vi "POST_sendNew_ServoStatus_toServo.vi"(11 "JSON_ServoStatus_fromClient":string) -> (0 "receivedBodyFromServo":string, 3 "receivedHeadersFromServo":string)   [LabVIEW 2024]
uses:
  <vilib>/httpClient/LabVIEWHTTPClient.lvlib
  DataTypes/OperationTypeForFunctionalGlobalVariable.ctl
  <vilib>/httpClient/POSTBuffer.vi
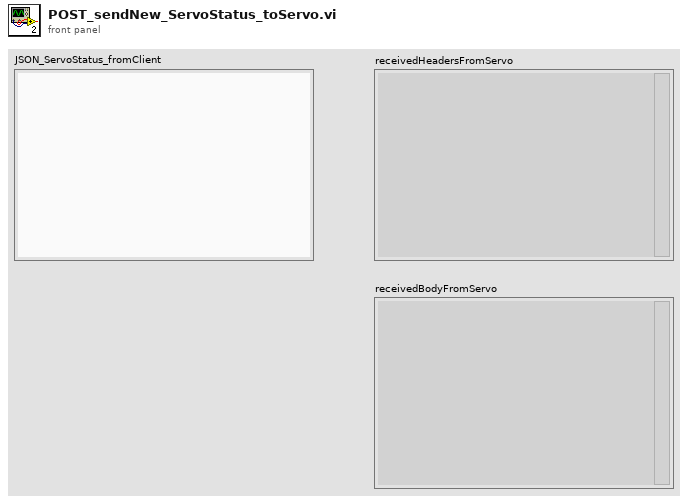
[diagram p1: front panel]
types:
  T1 = typedef "OperationTypeForFunctionalGlobalVariable.ctl" = enum16{"GET", "SET"}
  T2 = typedef "ServoConnectionParameters.ctl" = cluster{"host":string, "port":u16, "use_https":bool, "timeout_ms":u32, "base_url":string}
  T3 = typedef "LabVIEWHTTPClient.lvlib/ClientHandle.ctl" = refnum<k1>
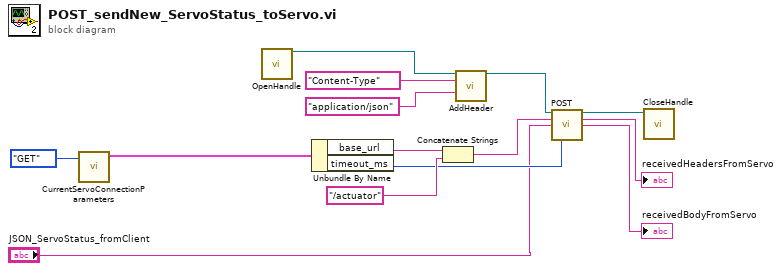
[diagram p0: block diagram]
diagram:
  n1 = call "CurrentServoConnectionParameters.vi"("Operation"=OperationTypeForFunctionalGlobalVariable."GET") -> ("Current Servo Connection Parameters"=w13:T2)  [unwired: 10 in]
  n2 = call <vilib>:"OpenHandle.vi"() -> ("client handle out"=w6:T3)  [unwired: 14 in, 1 out]
  n3 = Unbundle By Name(w13) -> ("base_url"=w14:string, "timeout_ms"=w4:u32)
  n4 = Concatenate Strings(w14, "/actuator" ("string")) -> (w10:string)
  n5 = call <vilib>:"AddHeader.vi"("client handle"=w6, "header"="Content-Type", "value"="application/json") -> ("client handle out"=w7:T3)  [unwired: 11 in, 1 out]
  n6 = call-poly <vilib>:"POST.vi"("client handle"=w7, "url"=w10, "buffer"="JSON_ServoStatus_fromClient", "timeout (10000)"=w4) -> ("client handle out"=w5:refnum<k1>, "headers"=→"receivedHeadersFromServo":string, "body"=→"receivedBodyFromServo":string)  [unwired: 8 in, 1 out]
  n7 = call <vilib>:"CloseHandle.vi"("client handle"=w5) -> ()  [unwired: 14 in, 1 out]
